vi "GetWindowAspectRatio.vi"(8 "No Error":errorcluster, 11 "Window [SDL_Window *]":i64 format="%.0x") -> (0 "Error Out":errorcluster, 2 "Max Aspect":sgl, 3 "Min Aspect":sgl)   [LabVIEW 2026, in "SDL3.lvlib" / "Video.lvlib"]
doc: "<B>Summary</B>\nGet the size of a window's client area."
uses:
  Video.lvlib
  <vilib>/Utility/error.llb/Error Cluster From Error Code.vi
  Error/Error.lvlib
  Lib/SDL3.dll
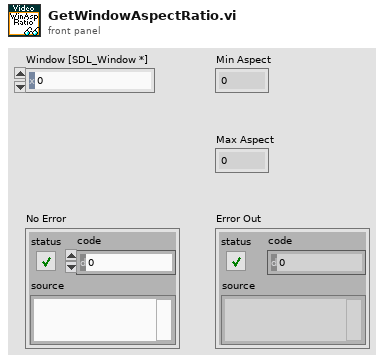
[diagram p1: front panel]
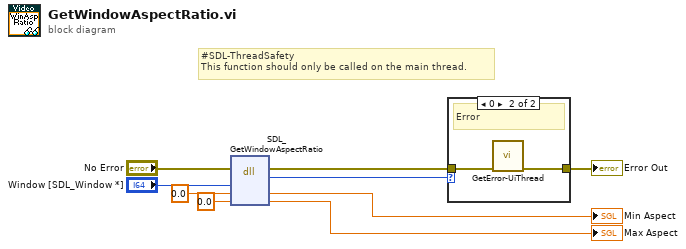
[diagram p0: block diagram]
diagram:
  # "#SDL-ThreadSafety\nThis function should only be called on the main thread."
  n1 = dll-call lib="C:/Users/saukko/Dev/LV-SDL3/Sources/SDL3/Lib/SDL3.*" fn="SDL_GetWindowAspectRatio"(error in="No Error", "window"="Window [SDL_Window *]", "min_aspect"=sgl 0.0, "max_aspect"=sgl 0.0) -> (error out=w4:errorcluster, "return type"=w3:i32, "min_aspect"=→"Min Aspect":sgl, "max_aspect"=→"Max Aspect":sgl)  [unwired: 3 in, 1 out]
  n2 = case shown="0" w3 {
    tunnel: w4 -> [w10 w12]
    tunnel: [w10 w11] -> w8
    frame Default {
      # "Ok"
    }
    frame 0 {
      # "Error"
      n3 = call "GetError-UiThread.vi"("No Error"=w12) -> ("error out"=w11:errorcluster)  [unwired: 10 in]
    }
  }
  "Error Out" <- w8
